vi "ParametersGlobal.vi"() -> ()   [LabVIEW 2019]
uses:
  <vilib>/vision/Image Controls.llb/IMAQ Image.ctl
  StimulusObject.lvclass
  <vilib>/userDefined/High Color/IMAQdx.ctl
panel:
  in  "PureGreenExposureTime":i32
  in  "RedBluePatternRepeat":i32
  in  "BlueLEDCurrent":u8
  in  "RedLEDCurrent":u8
  in  "GreenLEDCurrent":u8
  in  "BlueExposureTime":i32
  in  "RedExposureTime":i32
  in  "GreenExposureTime":i32
  in  "TC Zero XY values (Camera Pixels)":i32[][](array[numeric])
  in  "CalibrationBinaryThresholdLevel (out of 255)":dbl
  in  "Projector Camera Calibration Original":T1
  in  "Calibration Projector Dot Radius (camera pixel)":dbl
  in  "Spatial Calibration Camera Step Size (camera pixel)":dbl
  in  "Calibration Projector Dot Radius (projector pixel)":i32
  in  "Previous Camera Calibration Paper Points":cluster{"X":dbl, "Y":dbl}[](array[cluster])
  in  "Projector Calibration Points":cluster{"X":dbl, "Y":dbl}[](array[cluster])
  in  "Max Spatial Correction (camera pixel)":dbl
  in  "Previous Camera Calibration Particle Stats":dbl[][](array[numeric])
  in  "Tracking Max Backwards Time (Camera Frames)":i32
  in  "Stimulus Blue Power To Red Power Ratio":sgl
  in  "avgPowerBlue at 255 (wW/mm^2)":sgl
  in  "avgPowerRed at 255 (wW/mm^2)":sgl
  in  "avgPowerGreen at 255 (wW/mm^2)":sgl
  in  "Remote Path":string
  in  "Cluster IP Address":string="128.112.172.157"
  in  "Number of Buffer Images":i32=100
  in  "IMAQdx Session":T2="cam2"
  in  "Experiment Folder":string
  in  "Data Folder":string
  in  "Experimental Duration (Frames)":i32
  in  "Tracking Max Mature Tracks":i16
  in  "TC One XY values (Projector Pixels)":i32[][](array[numeric])
  in  "TC Zero XY values (Projector Pixels)":i32[][](array[numeric])
  in  "Stimulus Example Object":refnum<class "StimulusObject.lvclass">
  in  "Tracking Mature Time (Camera Frames)":i32
  in  "Tracking Centerline Points Count":i32
  in  "ParpoolTempIMAQArray":T1[](array[typedef])
  in  "ParpoolBinaryIMAQArray":T1[](array[typedef])
  in  "ParpoolOriginalIMAQArray":T1[](array[typedef])
  in  "Tracking Smoothing Window (Camera Frames)":i32
  in  "Projector Camera Calibration Image":T1
  in  "Camera Calibration Image":T1
  in  "Behavior Parallel Pool Count":i32
  in  "Tracking Worm Box Half Size (Camera Pixels)":i32
  in  "Tracking Max Worm Displacement (Camera Pixels/frame)":dbl
  in  "Tracking Max Worm Area (Camera Pixels^2)":dbl
  in  "Tracking Min Worm Area (Camera Pixels^2)":dbl
  in  "Tracking Max Area Change (Camera Pixels^2)":dbl
  in  "Tracking Max Blob Count":i32
  in  "Tracking Binary Threshold Level":sgl
  in  "Stimulus Buffer Size":i32
  in  "Tracking Memory Preallocation Size":i32
  in  "Camera Frame Rate (frames/s)":sgl
  in  "Initial Median Filter Aquisition Time (s)":dbl
  in  "Median Filter Update Time (ms)":i32
  in  "Number of Median Filter Images":i32
  in  "Projector Pixel to mm Conversion":sgl
  in  "Camera Pixel to mm Conversion":sgl
  in  "FW Worm Length s.d. (mm)":dbl
  in  "FW Worm Length mean (mm)":dbl
  in  "FW Initial Speed s.d. (mms/s)":dbl
  in  "FW Initial Speed mean (mms/s)":dbl
  in  "FW Speed change s.d. (mm/s/s)":dbl
  in  "FW Heading change s.d. (rad/s/s)":dbl
  in  "Image Width (camera pixel)":i32
  in  "Image Height (camera pixel)":i32
  in  "FW Poisson lambda":dbl
  in  "FW Max Faux Worm Count":i32
  in  "TC Dot Radius (Camera Pixels)":i32
  in  "TC Number of Other Bits Encoded":i32
  in  "TC One XY values (Camera Pixels)":i32[][](array[numeric])
  in  "TC Number of Time Bits Encoded":i32
  in  "TC Dot Radius (Projector Pixels)":i32
  in  "TC Zone Margin (Camera Pixels)":i32
  in  "TC Zone Radius (Camera Pixels)":i32
  # "Temporal Calibration"
  # "Faux Worm Drawing"
  # "Tracking"
  # "for expected number of worms\nto be added per round of adding"
  # "Camera and Projector Settings"
  # "Median Filtering"
  # "Paths"
  # "Stimulus Generation"
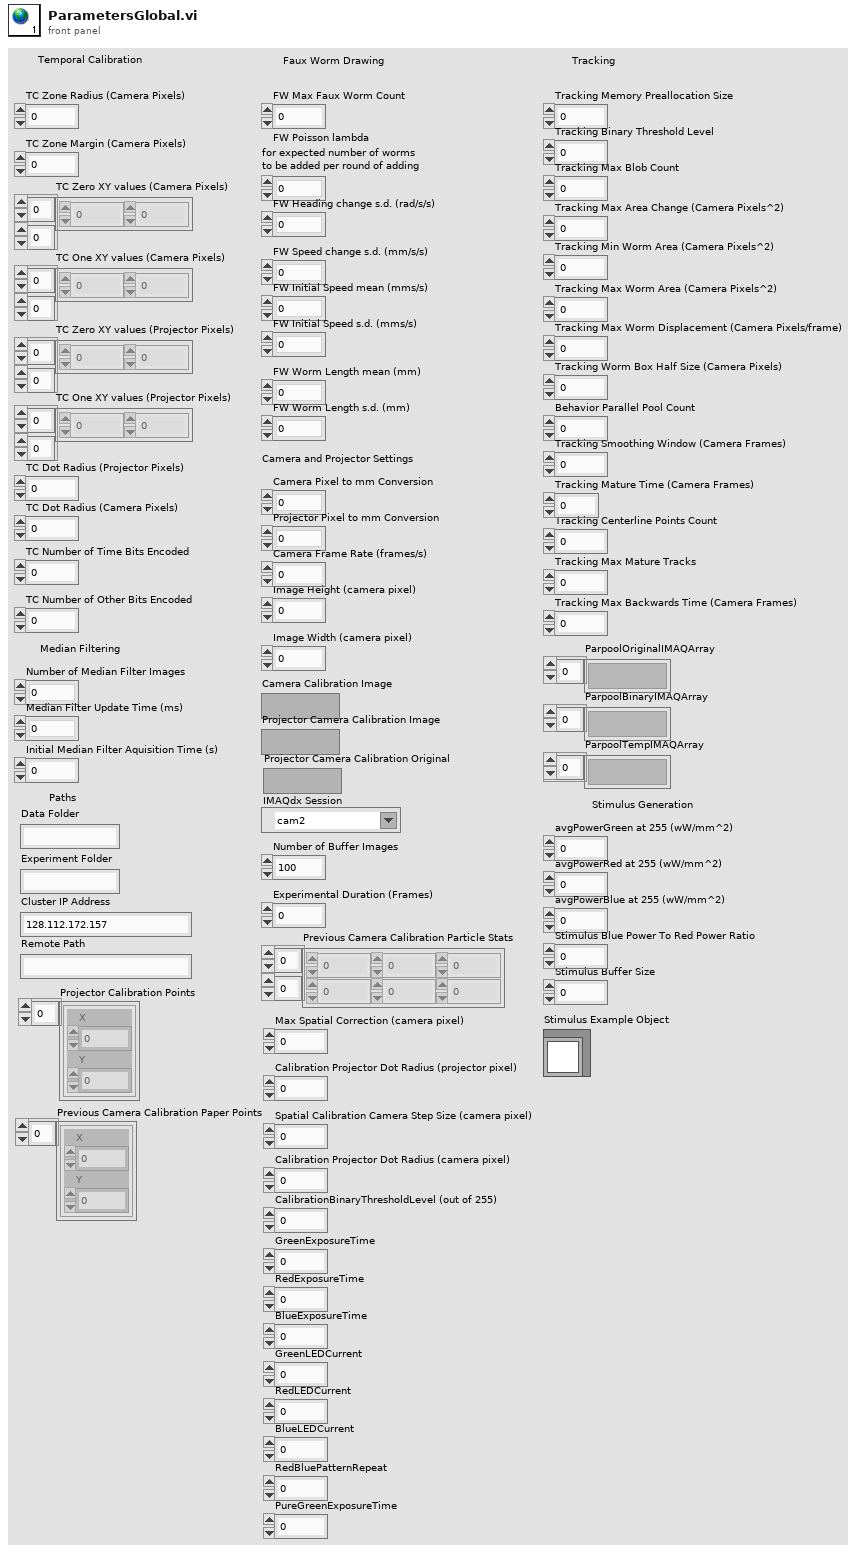
[diagram p1: front panel]
types:
  T1 = typedef "IMAQ Image.ctl" = refnum<image>
  T2 = typedef "IMAQdx.ctl" = refnum<k21>
diagram:
